vi "TP_Enqueue.vi"(8 "error in":errorcluster, 9 "Paras":variant, 10 "CMD":string, 11 "name":string="UI") -> (0 "error out":errorcluster)   [LabVIEW 2012]
uses:
  TP_Message data.ctl
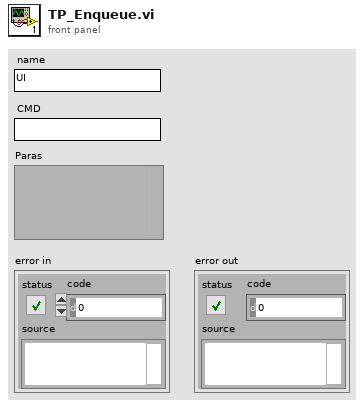
[diagram p1: front panel]
types:
  T1 = typedef "TP_Message data.ctl" = cluster{"CMD":string, "Paras":variant}
  T2 = enum16{"Create Queue", "Get Queue", "Destory Queue"}
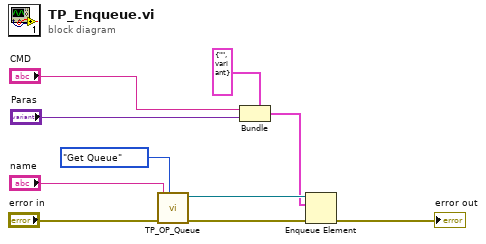
[diagram p0: block diagram]
diagram:
  n1 = call "TP_OP_Queue.vi"("OP_Queue (get queue)"=T2."Get Queue", "error in"="error in", "name (unnamed)"="name") -> ("error out"=w3:errorcluster, "queue out"=w8:refnum<queue>)  [unwired: 7 in]
  n2 = Bundle(cluster=T1 {"CMD"="", "Paras"=variant} ("element"), "CMD"="CMD", "Paras"="Paras") -> (w4:T1)
  n3 = Enqueue Element(queue=w8, element=w4, error in (no error)=w3) -> (error out=→"error out":errorcluster)  [unwired: 1 in, 2 out]
